vi "Add segment number to property name.vi"(0 "Fcurve segment.nb":u8, 1 "Property Name":string[](array[string])) -> (14 "Segment_#_propertyName":string[](array[string]))   [LabVIEW 2019, in "metadata.lvclass"]
uses:
  metadata.lvclass
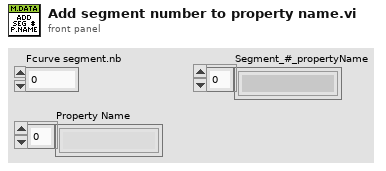
[diagram p1: front panel]
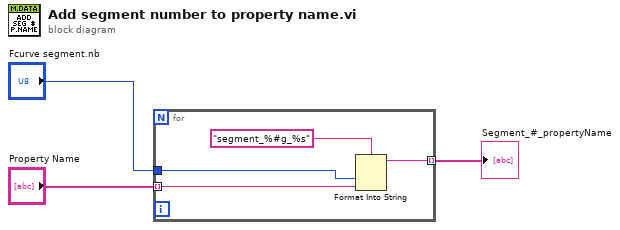
[diagram p0: block diagram]
diagram:
  n1 = for {
    tunnel: "Property Name" -> [w5] mode=indexing
    tunnel: "Fcurve segment.nb" -> [w6]
    tunnel: [w4] -> w3 mode=indexing
    n2 = Format Into String(format string="segment_%#g_%s", w6, w5) -> (resulting string=w4:string)  [unwired: 2 in, 1 out]
  }
  "Segment_#_propertyName" <- w3
